vi "Write Conf File Path.vi"(10 "Conf File Path":path, 11 "Generic Test Stand in":refnum<class "Generic Test Stand.lvclass">) -> (3 "Generic Test Stand out":refnum<class "Generic Test Stand.lvclass">)   [LabVIEW 2019, in "Generic Test Stand.lvclass"]
uses:
  Generic Test Stand.lvclass
  Generic Test Stand.lvclass/Generic Test Stand.ctl
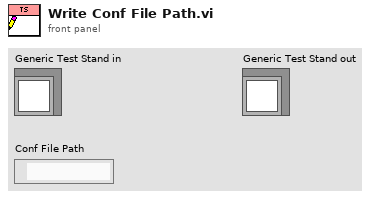
[diagram p1: front panel]
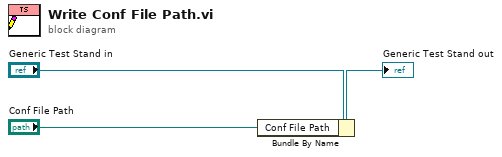
[diagram p0: block diagram]
diagram:
  n1 = Bundle By Name(cluster="Generic Test Stand in", "Conf File Path"="Conf File Path") -> (→"Generic Test Stand out":refnum<class "Generic Test Stand.lvclass">)
